vi "Polling.vi"(4 "Cycle RFID Enable":bool=TRUE, 5 "Stn_No":i32, 6 "Enable?":bool=TRUE, 7 "RFID Scanned":string, 8 "error in (no error)":errorcluster, 10 "STATUS":i32, 11 "Ref in":T1={"MS SQL Connection"=refnum, "UDL File"=path "", "Time"="", "DCODE"="", "WIP+1"=0, "MC No?"=0, "POKAYOKE?"=FALSE, "Expected Result"="", "Result [Status]"="", "Clock"=0.0, "RFID"="", "WIP Queue"=refnum, "TS Parameter"={"ProfitCenterCode"="", "LineCode"="", "WorkOrderNumber"="", "Model"="", "Model_with_Prefix"="", "VendorCode"="", "SetParameterDateCode"="", "PokaYoke"=0, "Target"=1, "Live_DateCode"="", "CustomerPartNumber"="", "Hand"="", "sBarcode"=FALSE, "FCA"=0, "Ent_Stamp"=timestamp(0 s since 1904-01-01), "STS_CD"=0.0}, "Data_Queue"=[], "RFID Serial No."=""} {"TS Parameter"."FCA" format="%01d"; "TS Parameter"."Target" min=1 max=100000; "TS Parameter"."PokaYoke" min=0 max=1}) -> (0 "error out":errorcluster, 2 "State Out":T4, 3 "Ref out":T1={"MS SQL Connection"=refnum, "UDL File"=path "", "Time"="", "DCODE"="", "WIP+1"=0, "MC No?"=0, "POKAYOKE?"=FALSE, "Expected Result"="", "Result [Status]"="", "Clock"=0.0, "RFID"="", "WIP Queue"=refnum, "TS Parameter"={"ProfitCenterCode"="", "LineCode"="", "WorkOrderNumber"="", "Model"="", "Model_with_Prefix"="", "VendorCode"="", "SetParameterDateCode"="", "PokaYoke"=0, "Target"=1, "Live_DateCode"="", "CustomerPartNumber"="", "Hand"="", "sBarcode"=FALSE, "FCA"=0, "Ent_Stamp"=timestamp(0 s since 1904-01-01), "STS_CD"=0.0}, "Data_Queue"=[], "RFID Serial No."=""} {"TS Parameter"."FCA" format="%01d"; "TS Parameter"."Target" min=1 max=100000; "TS Parameter"."PokaYoke" min=0 max=1})   [LabVIEW 2020]
uses:
  Controls/Station_Task.ctl
  Controls/TD SQL.ctl
  <vilib>/addons/database/Connection.llb/Conn ObjectReference.ctl
  Controls/WIP_State.ctl
  Controls/TS_Parameter.ctl
  MS SQL/MS_Global.vi
  <userlib>/_OpenG.lib/comparison/comparison.llb/Boolean Changed__ogtk.vi
  <vilib>/addons/database/NI_Database_API.lvlib
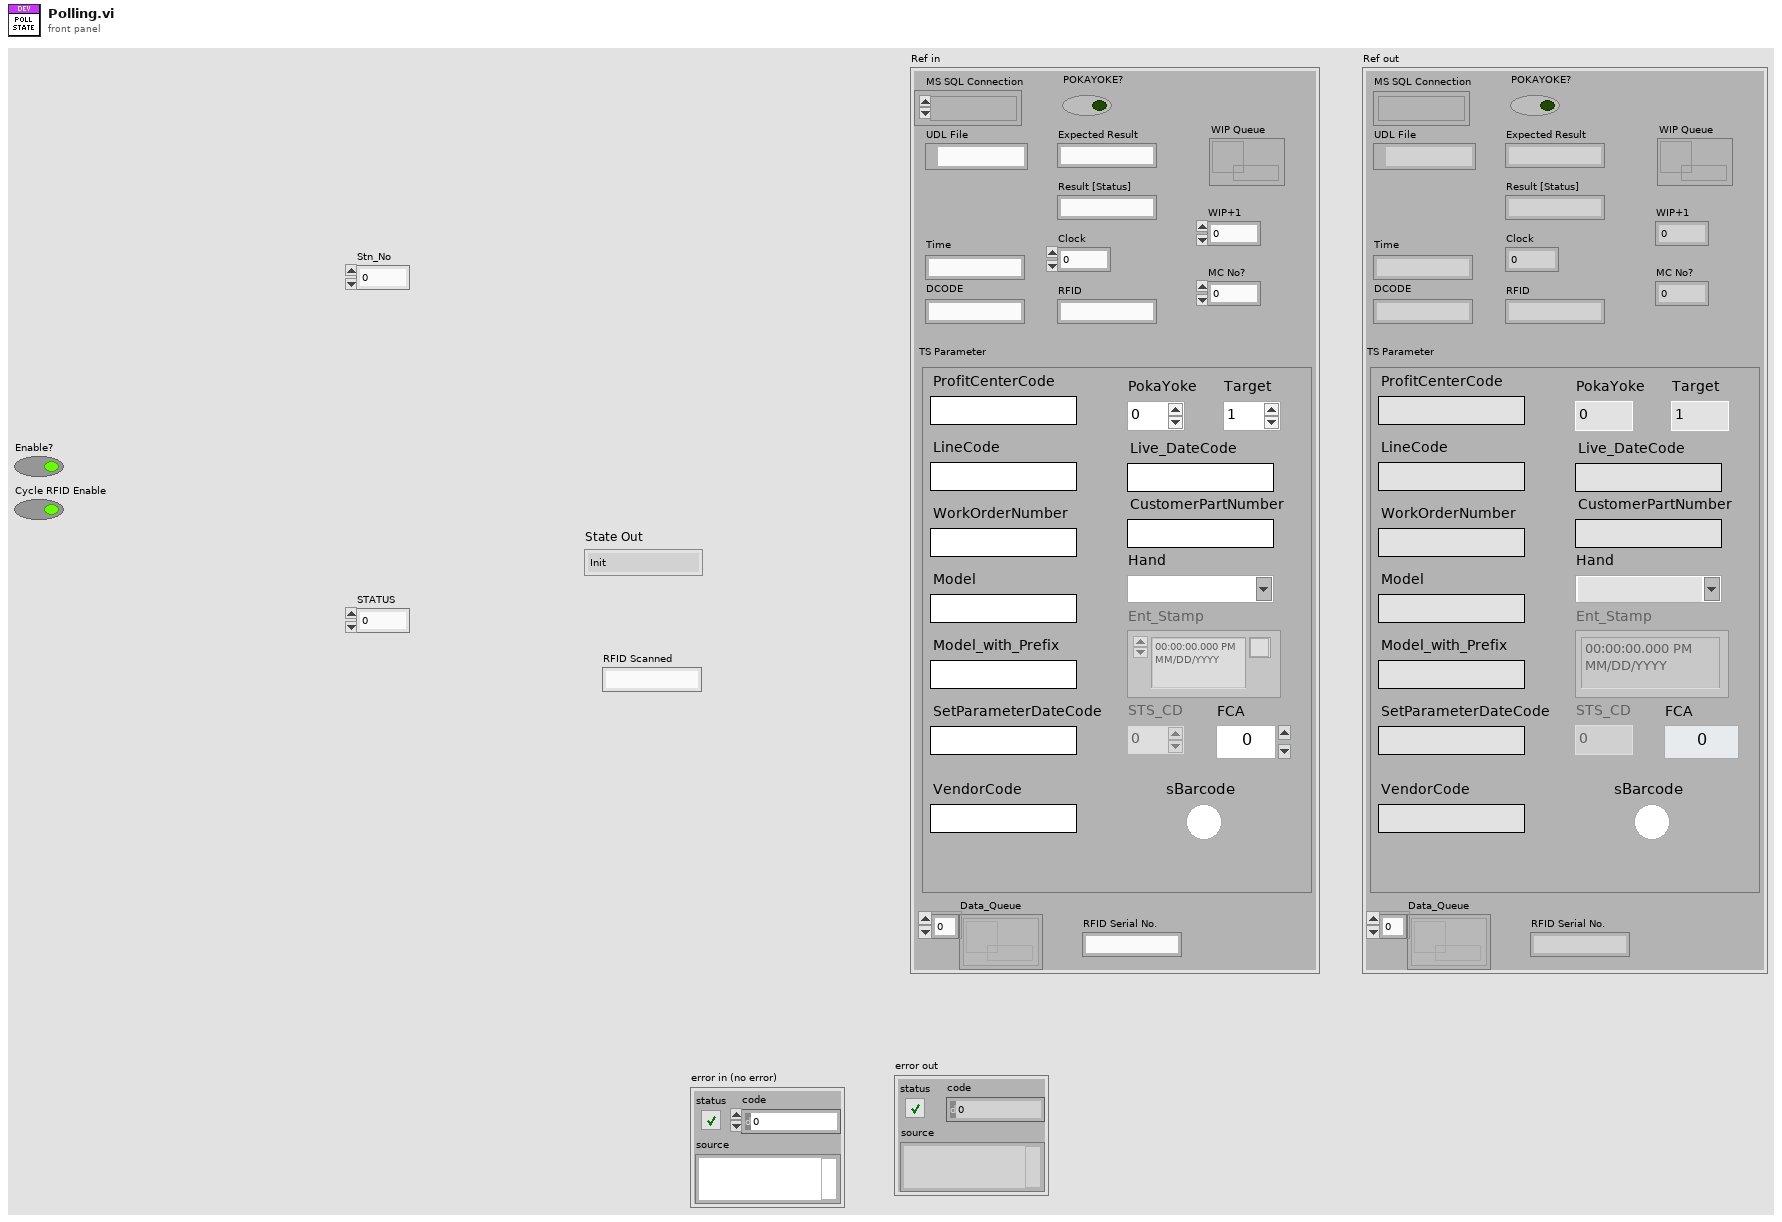
[diagram p1: front panel]
types:
  T1 = typedef "TD SQL.ctl" = cluster{"MS SQL Connection":T2, "UDL File":path, "Time":string, "DCODE":string, "WIP+1":i64, "MC No?":i32, "POKAYOKE?":bool, "Expected Result":string, "Result [Status]":string, "Clock":dbl, "RFID":string, "WIP Queue":refnum<queue>, "TS Parameter":T3, "Data_Queue":refnum<queue>[], "RFID Serial No.":string}
  T2 = typedef "NI_Database_API.lvlib/Conn ObjectReference.ctl" = refnum<k1>
  T3 = typedef "TS_Parameter.ctl" = cluster{"ProfitCenterCode":string, "LineCode":string, "WorkOrderNumber":string, "Model":string, "Model_with_Prefix":string, "VendorCode":string, "SetParameterDateCode":string, "PokaYoke":i32, "Target":i32, "Live_DateCode":string, "CustomerPartNumber":string, "Hand":string, "sBarcode":bool, "FCA":i32, "Ent_Stamp":timestamp, "STS_CD":dbl}
  T4 = typedef "Station_Task.ctl" = enum16{"Init", "Polling", "Check Bypass", "Check_Result", "get Barcode", "Pass", "Fail", "Check Data", "Log Data", "Idle_Alert", "DMS_Check", "FV_Check", "FV_View", "WRITE_RFID", "Exit"}
  T5 = typedef "Idle_Timer.ctl" = cluster{"OP10":T6, "OP20":T6, "OP30":T6, "OP40":T6, "OP50":T6, "OP60":T6}
  T6 = typedef "Idle_Timer_disp.ctl" = dbl
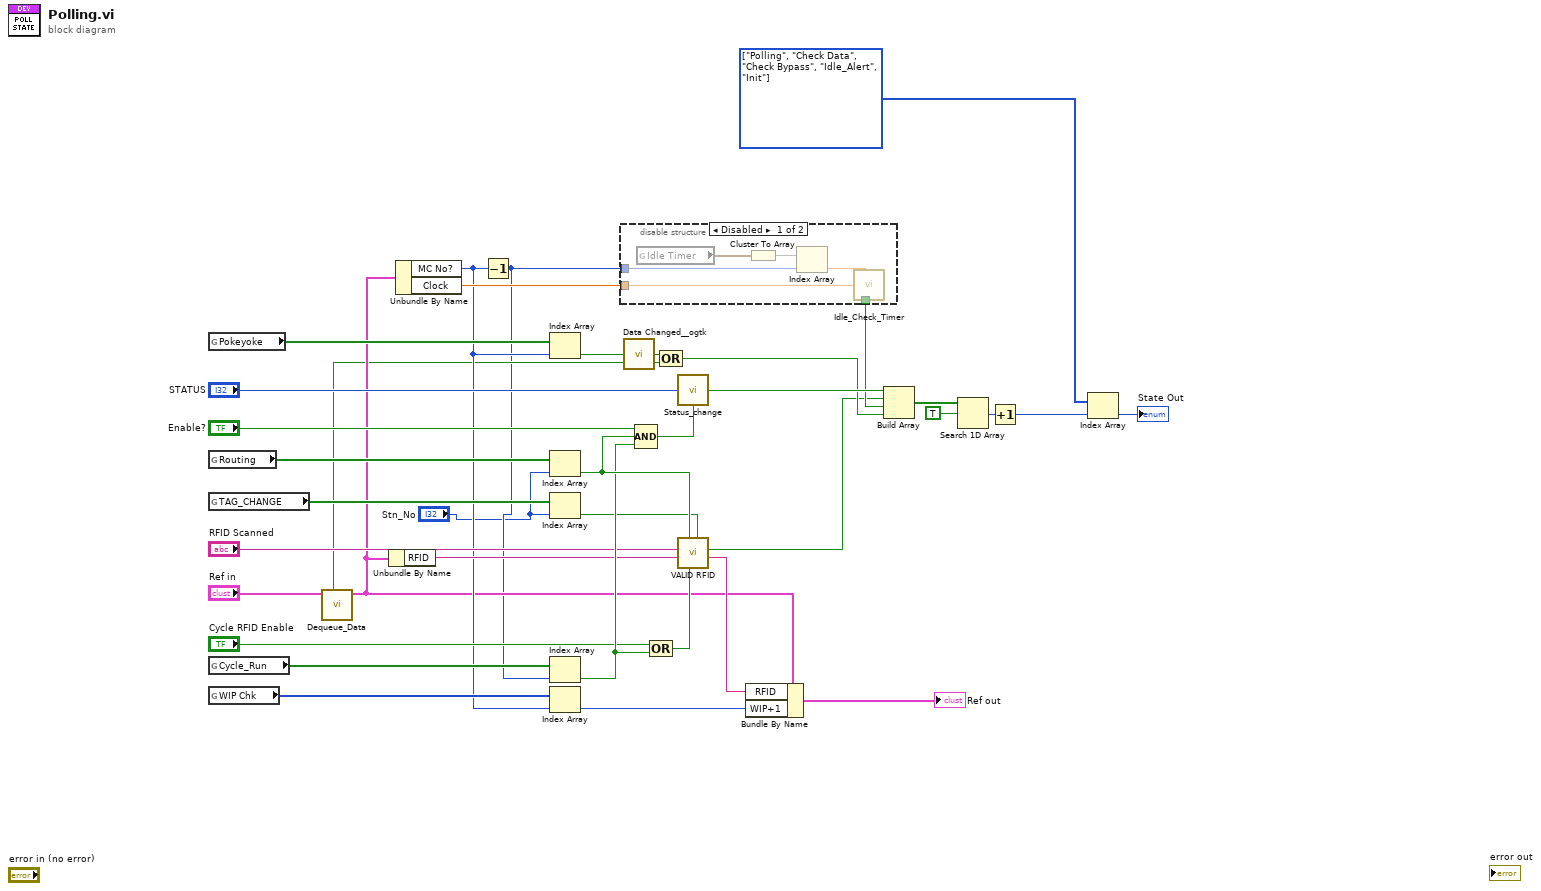
[diagram p0: block diagram]
diagram:
  w31 = T4[] [enum."Polling", enum."Check Data", enum."Check Bypass", enum."Idle_Alert", enum."Init"] items=["Init", "Polling", "Check Bypass", "Check_Result", "get Barcode", "Pass", "Fail", "Check Data", "Log Data", "Idle_Alert", "DMS_Check", "FV_Check", "FV_View", "WRITE_RFID", "Exit"]
  n1 = global read "MS_Global.vi" "Pokeyoke"() -> (w25:bool[])
  n2 = global read "MS_Global.vi" "Routing"() -> (w23:bool[])
  n3 = global read "MS_Global.vi" "TAG_CHANGE"() -> (w10:bool[])
  n4 = global read "MS_Global.vi" "Cycle_Run"() -> (w18:bool[])
  n5 = global read "MS_Global.vi" "WIP Chk"() -> (w8:i64[])
  n6 = call "Dequeue_Data.vi"("Ref in"="Ref in") -> ("Ref Out"=w4:T1, "Data Change"=w3:bool)  [unwired: 5 in, 2 out]
  n7 = Unbundle By Name(w4) -> ("RFID"=w16:string)
  n8 = Unbundle By Name(w4) -> ("MC No?"=w6:i32, "Clock"=w26:dbl)
  n9 = Decrement(x=w6) -> (x-1=w2:i32)
  n10 = Index Array(array=w25, index=w6) -> (element=w24:bool)
  n11 = Index Array(array=w23, index="Stn_No") -> (element=w22:bool)
  n12 = Index Array(array=w10, index="Stn_No") -> (element=w9:bool)
  n13 = Index Array(array=w18, index=w2) -> (element=w17:bool)
  n14 = Index Array(array=w8, index=w6) -> (element=w7:i64)
  n15 = disable-structure shown="Disabled" {
    disable-tunnel: [w43 _] -> w35
    disable-tunnel: w26 -> [w42 _]
    disable-tunnel: w2 -> [w38 _]
    frame Disabled {
      n16 = global read "MS_Global.vi" "Idle Timer"() -> (w41:T5)
      n17 = Cluster To Array(cluster=w41) -> (array=w40:T6[])
      n18 = Index Array(array=w40, index=w38) -> (element=w39:T6)
      n19 = call "Idle_Check_Timer.vi"("Time Interval"=w39, "Previous Time In (Sec)"=w42) -> ("Idle?"=w43:bool)  [unwired: 4 in, 1 out]
    }
    frame Enabled {
    }
  }
  n20 = call-poly <userlib>:"Data Changed__ogtk.vi"("Boolean"=w24) -> ("Changed"=w33:bool)
  n21 = Compound Arithmetic op=AND("Enable?", w22, w17) -> (w20:bool)
  n22 = Compound Arithmetic op=OR("Cycle RFID Enable", w17) -> (w12:bool)
  n23 = Compound Arithmetic op=OR(w33, w3) -> (w34:bool)
  n24 = call "Status_change.vi"("Routing"=w20, "OP10B STATUS"="STATUS") -> ("Status Change"=w37:bool)  [unwired: 2 in]
  n25 = call "VALID RFID.vi"("Tag Change"=w9, "Cycle Start"=w12, "Bypass?"=w22, "RFID-1"=w16, "RFID"="RFID Scanned") -> ("RFID OUT"=w15:string, "CHANGED?"=w14:bool)  [unwired: 5 in]
  n26 = Bundle By Name(cluster=w4, "RFID"=w15, "WIP+1"=w7) -> (→"Ref out":T1)
  n27 = Build Array(w37, w14, w35, w34) -> (w27:bool[])
  n28 = Search 1D Array(1D array=w27, element=TRUE) -> (index of element=w29:i32)  [unwired: 1 out]
  n29 = Increment(x=w29) -> (x+1=w30:i32)
  n30 = Index Array(array=w31, index=w30) -> (element=→"State Out":T4)
